vi "test Write Controls to INI.vi"() -> ()   [LabVIEW 2017]
uses:
  <vilib>/Utility/config.llb/NI_LVConfig.lvlib
panel:
  in  "$Numeric 5":dbl
  in  "Numeric 4":dbl
  in  "_Numeric 3":dbl
  in  "Numeric 2":dbl
  in  "*Numeric":dbl
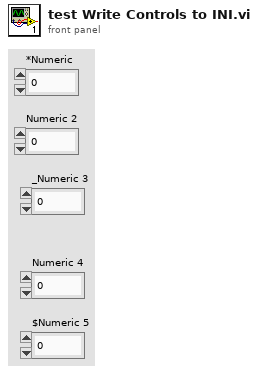
[diagram p1: front panel]
types:
  T1 = typedef "NI_LVConfig.lvlib/Config Data RefNum.ctl" = refnum<k1>
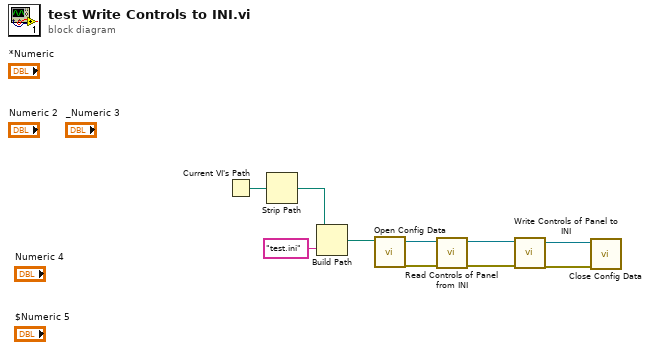
[diagram p0: block diagram]
diagram:
  n1 = Current VI's Path() -> (path=w8:path)
  n2 = Strip Path(path=w8) -> (stripped path=w1:path)  [unwired: 1 out]
  n3 = Build Path(base path=w1, name or relative path="test.ini") -> (appended path=w6:path)
  n4 = call <vilib>:"Open Config Data.vi"("configuration file path"=w6) -> ("error out"=w4:errorcluster, "refnum"=w5:T1)  [unwired: 8 in, 1 out]
  n5 = call "Read Controls of Panel from INI.vi"("error in (no error)"=w4, "refnum"=w5) -> ("error out"=w2:errorcluster, "refnum out"=w3:T1)  [unwired: 8 in]
  n6 = call "Write Controls of Panel to INI.vi"("error in (no error)"=w2, "refnum"=w3) -> ("error out"=w9:errorcluster, "refnum out"=w10:T1)  [unwired: 8 in]
  n7 = call <vilib>:"Close Config Data.vi"("error in (no error)"=w9, "refnum"=w10) -> ()  [unwired: 8 in, 2 out]
